vi "Logger Daemon.vi"(8 "Error In":errorcluster, 11 "TDMS Log In":refnum<class "TDMS Logger.lvclass">) -> ()   [LabVIEW 2019, in "TDMS Logger.lvlib" / "TDMS Logger.lvclass"]
uses:
  TDMS Logger.lvclass
  TDMS Logger.lvclass/TDMS Logger.ctl
  _Typedefs/Log Action.ctl
  _Typedefs/Log Message.ctl
  _Typedefs/Data Type.ctl
  <vilib>/Utility/High Resolution Relative Seconds.vi
  <vilib>/Rock Robotics/Network Tables/NT Write Value.vi
  <vilib>/Rock Robotics/Network Tables/NT Write Numeric Array.vi
  <vilib>/Rock Robotics/Network Tables/NT Write String Array.vi
  <vilib>/Rock Robotics/Network Tables/NT Write Variant.vi
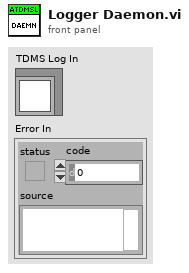
[diagram p1: front panel]
types:
  T1 = typedef "TDMS Logger.lvlib/TDMS Logger.lvclass/Log Action.ctl" = enum16{"Handle Old Files", "Status Update", "Stop", "Log Data", "Initialize"}
  T2 = typedef "TDMS Logger.lvlib/TDMS Logger.lvclass/Log Message.ctl" = cluster{"Log Action":T1, "Variant":variant, "Data Type":T3, "Group Name":string, "Channels Names":string[]}
  T3 = typedef "TDMS Logger.lvlib/TDMS Logger.lvclass/Data Type.ctl" = enum16{"I16", "I8", "String", "U16", "U8", "Waveform", "Double", "Single"}
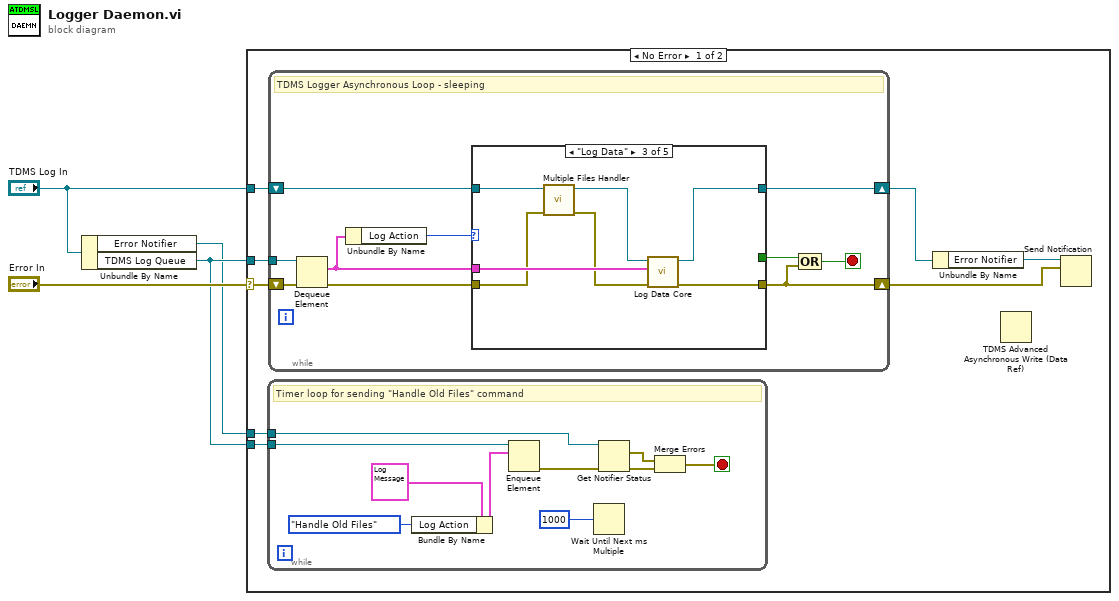
[diagram p0: block diagram]
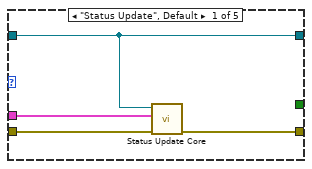
[diagram p2: hidden frame]
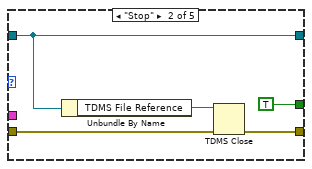
[diagram p3: hidden frame]
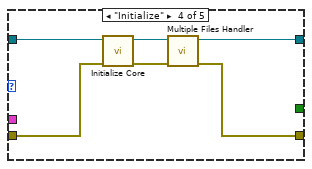
[diagram p4: hidden frame]
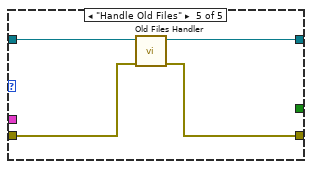
[diagram p5: hidden frame]
diagram:
  n1 = Unbundle By Name("TDMS Log In") -> ("Error Notifier"=w1:refnum<notifier>, "TDMS Log Queue"=w2:refnum<queue>)
  n2 = case shown="No Error" "Error In" {
    selector: "Error In" -> [w11 _]
    tunnel: "TDMS Log In" -> [w12 _]
    tunnel: w2 -> [w10 _]
    tunnel: w2 -> [w6 _]
    tunnel: w1 -> [w5 _]
    frame No Error {
      n3 = while {
        tunnel: w6 -> [w58]
        tunnel: w5 -> [w52]
        stop <- w49 stop-if-true
        # "Timer loop for sending \"Handle Old Files\" command"
        n4 = Bundle By Name(cluster=T2 {"Log Action"=enum."Stop", "Variant"=variant, "Data Type"=enum."String", "Group Name"="", "Channels Names"=[]} ("element"), "Log Action"=Log_Action."Handle Old Files") -> (w54:T2)
        n5 = Enqueue Element(queue=w58, element=w54) -> (error out=w53:errorcluster)  [unwired: 2 in, 2 out]
        n6 = Wait Until Next ms Multiple(millisecond multiple=u32 1000) -> ()  [unwired: 1 out]
        n7 = Get Notifier Status(notifier=w52, error in (no error)=w53) -> (current notification=w50:errorcluster, error out=w51:errorcluster)  [unwired: 3 out]
        n8 = Merge Errors(w50, w51) -> (w49:errorcluster)
      }
      n9 = while {
        shift-right: [w16] -> w9
        shift-left: w12 -> [w18]
        tunnel: w10 -> [w21]
        shift-right: [w15] -> w7
        shift-left: w11 -> [w22]
        stop <- w19 stop-if-true
        # "TDMS Logger Asynchronous Loop - sleeping"
        n10 = Dequeue Element(queue=w21, error in (no error)=w22) -> (element=w14:T2, error out=w17:errorcluster)  [unwired: 1 in, 2 out]
        n11 = Unbundle By Name(w14) -> ("Log Action"=w13:T1)
        n12 = case shown="\"Log Data\"" w13 {
          tunnel: w14 -> [w26 _ w38 _ _]
          tunnel: w17 -> [w24 w30 w36 w39 w46]
          tunnel: [w23 w29 w35 w42 w45] -> w15
          tunnel: [_ TRUE _ _ _] -> w20
          tunnel: [w25 w28 w34 w43 w47] -> w16
          tunnel: w18 -> [w25 w28 w37 w44 w48]
          frame "Status Update", Default {
            n13 = call "Status Update Core.vi"("Error In"=w24, "Log Message"=w26, "TDMS Log In"=w25) -> ("Error Out"=w23:errorcluster)  [unwired: 8 in]
          }
          frame "Stop" {
            n14 = Unbundle By Name(w28) -> ("TDMS File Reference"=w27:refnum<k34>)
            n15 = TDMS Close(8:w30, 11:w27) -> (0:w29:errorcluster)  [unwired: 1 out]
          }
          frame "Log Data" {
            n16 = call "Multiple Files Handler.vi"("Error In"=w36, "TDMS Log"=w37) -> ("Error Out"=w32:errorcluster, "TDMS Log Out"=w33:refnum<class "TDMS Logger.lvclass">)  [unwired: 8 in]
            n17 = call "Log Data Core.vi"("Error In"=w32, "Log Message"=w38, "TDMS Log In"=w33) -> ("Error Out"=w35:errorcluster, "TDMS Log Out"=w34:refnum<class "TDMS Logger.lvclass">)  [unwired: 7 in]
          }
          frame "Initialize" {
            n18 = call "Initialize Core.vi"("Error In"=w39, "TDMS Log In"=w44) -> ("Error Out"=w40:errorcluster, "TDMS Log Out"=w41:refnum<class "TDMS Logger.lvclass">)  [unwired: 8 in]
            n19 = call "Multiple Files Handler.vi"("Error In"=w40, "TDMS Log"=w41) -> ("Error Out"=w42:errorcluster, "TDMS Log Out"=w43:refnum<class "TDMS Logger.lvclass">)  [unwired: 8 in]
          }
          frame "Handle Old Files" {
            n20 = call "Old Files Handler.vi"("Error In"=w46, "TDMS Log"=w48) -> ("Error Out"=w45:errorcluster, "TDMS Log"=w47:refnum<class "TDMS Logger.lvclass">)  [unwired: 8 in]
          }
        }
        n21 = Compound Arithmetic op=OR(w20, w15) -> (w19:bool)
      }
      n22 = Unbundle By Name(w9) -> ("Error Notifier"=w8:refnum<notifier>)
      n23 = TDMS Advanced Asynchronous Write (Data Ref)() -> ()  [unwired: 4 in, 2 out]
      n24 = Send Notification(notification=w7, notifier=w8) -> ()  [unwired: 1 in, 2 out]
    }
    frame Error {
    }
  }
